vi "Main-Scanner.vi"() -> ()   [LabVIEW 2015]
uses:
  <vilib>/Utility/miscctls.llb/LVPointTypeDef.ctl
  <vilib>/Utility/sysdir.llb/System Directory Type.ctl
  <vilib>/event_ctls.llb/eventvkey.ctl
  <vilib>/Utility/config.llb/Read Key (I32).vi
  <vilib>/Utility/config.llb/Read Key (Boolean).vi
  <vilib>/Utility/config.llb/Read Key (String).vi
  <vilib>/Utility/config.llb/Write Key (U32).vi
  <vilib>/Utility/config.llb/Write Key (String).vi
  <vilib>/Utility/config.llb/NI_LVConfig.lvlib
panel:
  out "작업자명-Ready":bool=TRUE caption="Ready"
  out "Log 경로":path
  in  "Log File":bool
  out "공정단계-Ready":bool=TRUE caption="Ready"
  out "공정선택-Ready":bool=TRUE caption="Ready"
  out "Info.":string
  out "Ready":bool
  in  "제품번호":string
  in  "작업자명":string
  in  "공정 선택-Lock":bool caption="Lock"
  in  "공정단계":u16(ring) items=["Start", "Pass", "Fail"]
  in  "공정 선택":u16(ring) items=["Battery Cal.", "Glue Printing", "Leak Test", "FTS Test", "Package"]
  out "Path":path caption="경로 복제"
  out "ms 타이머 값":u32=30688000
  out "스캔 문자 삭제":bool=TRUE
  out "스캔 문자 수신 종료":bool
  out "Buf":string
  out "스캔 대기":bool=TRUE
  out "스캔 입력":bool
  in  "종료":bool=TRUE
  # "Ver. 161007"
  # "스캔대상"
  # "PCBA/박스.파우치"
  # "스캐너"
  # "Digital Scanner\n* DS4308"
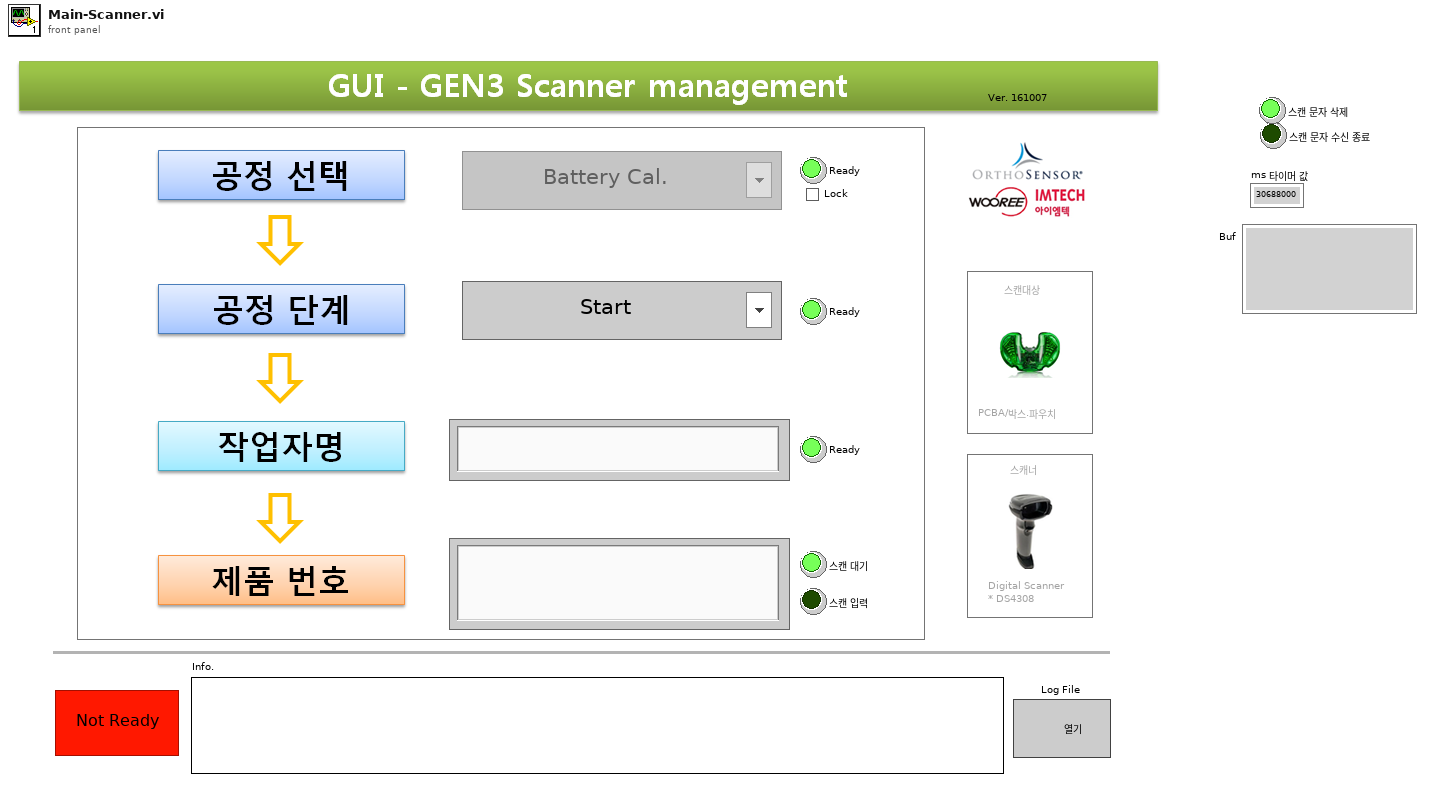
[diagram p1: front panel]
types:
  T1 = enum16{"Always On", "Always Off", "Off While Running"}
  T2 = typedef "LVPointTypeDef.ctl" = cluster{"Horizontal":i16, "Vertical":i16}
  T3 = enum8{"Enabled", "Disabled", "Disabled and Grayed Out"}
  T4 = typedef "eventvkey.ctl" = enum16{"ASCII", "Enter", "Return", "Shift", "Ctrl", "Alt", "Cmd", "Opt", "Caps", "NumLock", "Clear", "Break", "Up", "Down", "Left", "Right", "Insert", "Delete", "Home", "End", "PageUp", "PageDown", "Escape", "Help", "Pause", "ScrollLock", "F1", "F2", "F3", "F4", "F5", "F6", "F7", "F8", "F9", "F10", "F11", "F12", "F13", "F14", "F15", "F16", "F17", "F18", "F19", "F20", "F21", "F22", "F23", "F24", "Play", "VolumeUp", "VolumeDown", "Mute", "Two Byte Char"}
  T5 = enum16{"open", "replace", "create", "open or create", "replace or create", "replace or create with confirmation"}
  T6 = enum32{"invalid app kind", "Development System", "Run Time System", "Student Edition", "Embedded LabVIEW", "Evaluation", "Custom"}
  T7 = typedef "System Directory Type.ctl" = i32
  T8 = typedef "NI_LVConfig.lvlib/Config Data RefNum.ctl" = refnum<k1>
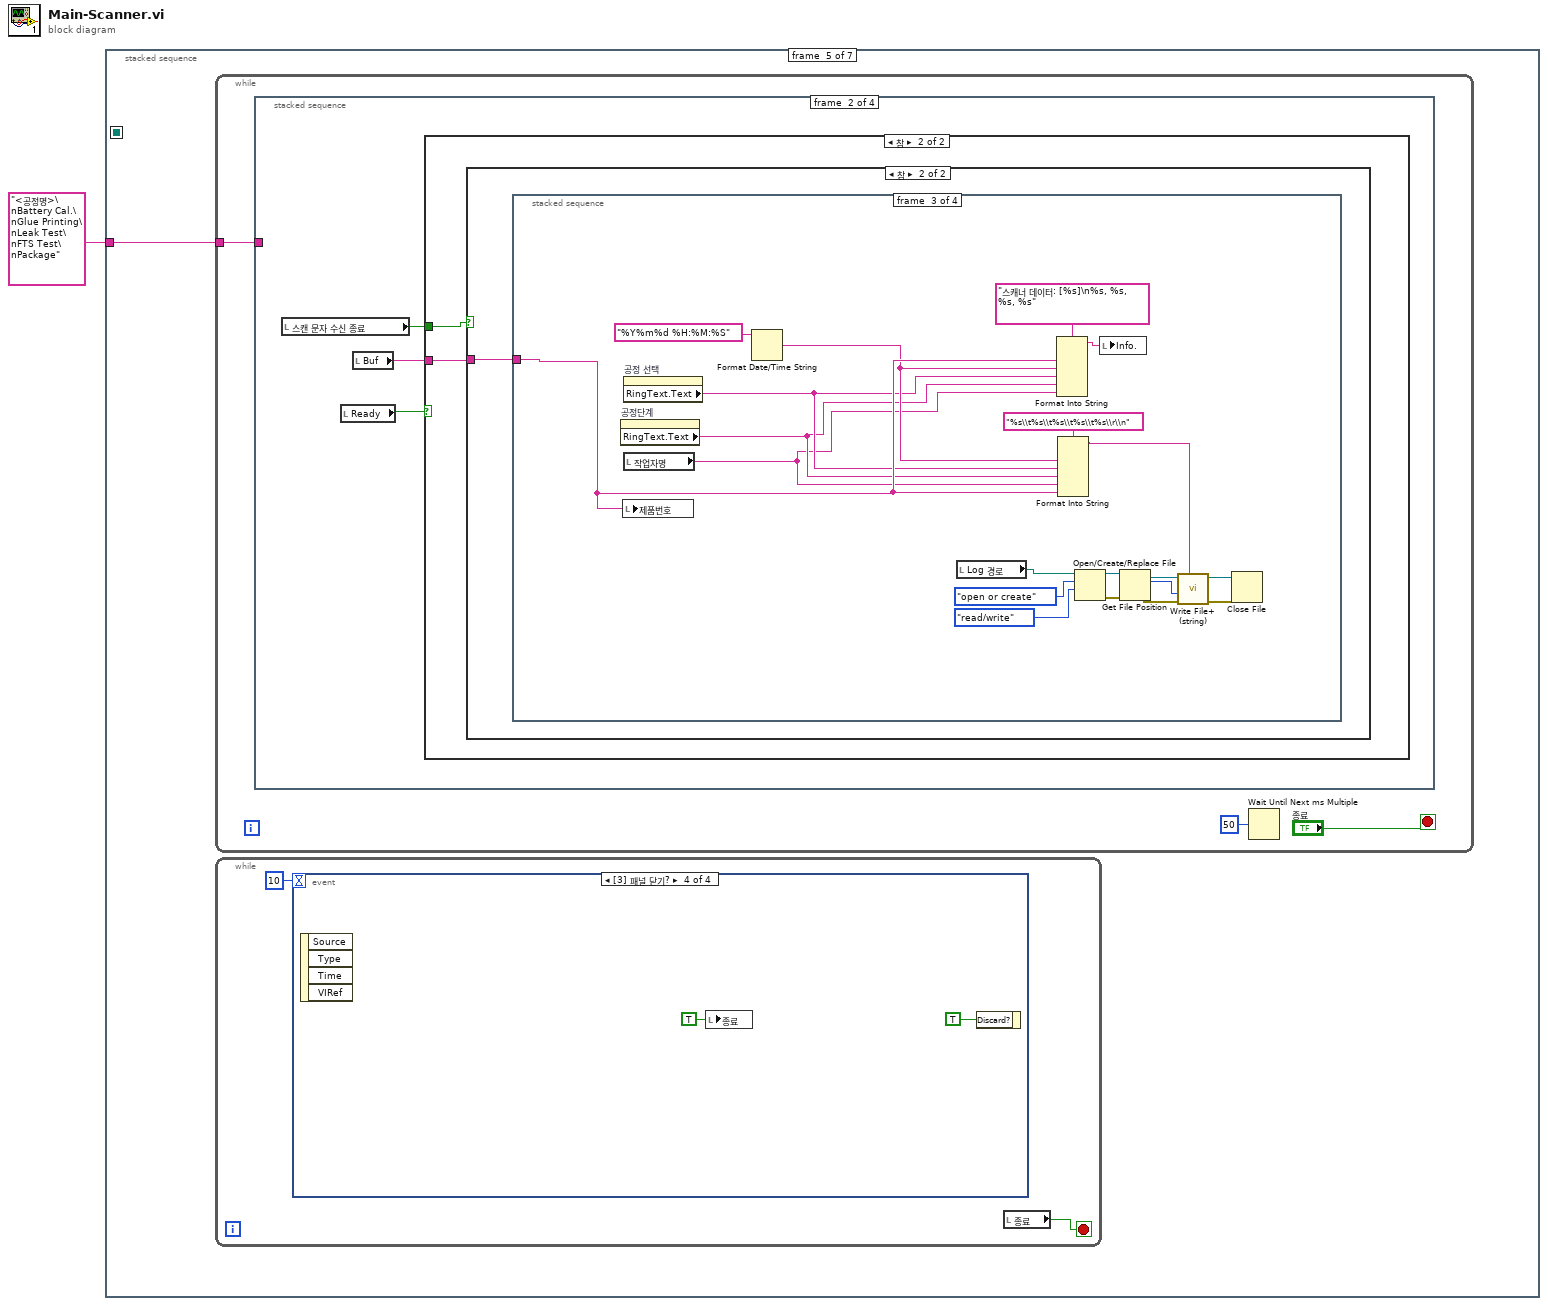
[diagram p0: block diagram]
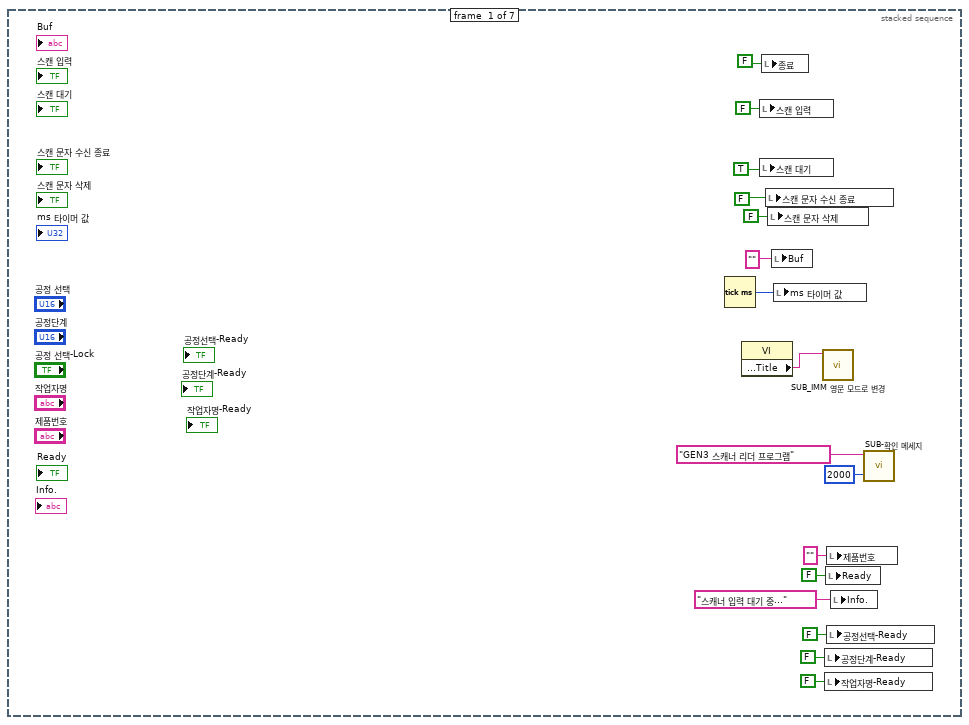
[diagram p2: hidden frame]
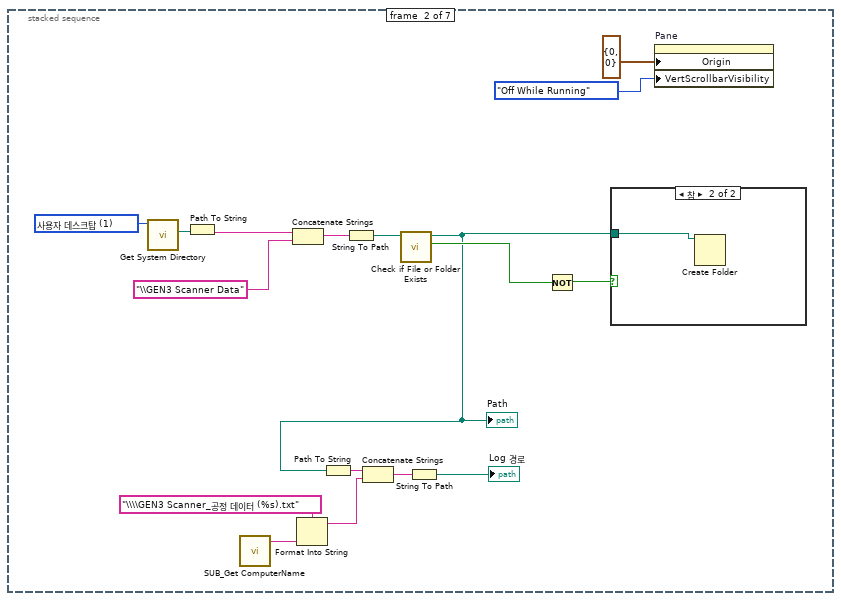
[diagram p3: hidden frame]
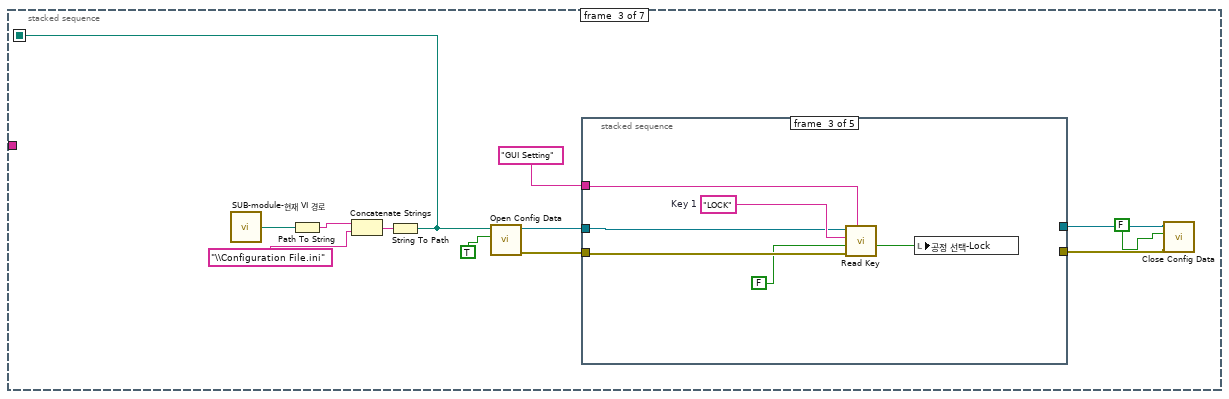
[diagram p5: hidden frame]
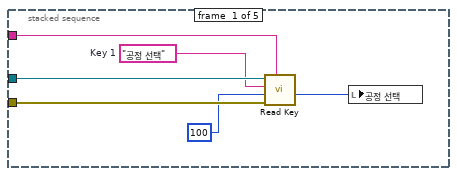
[diagram p6: hidden frame]
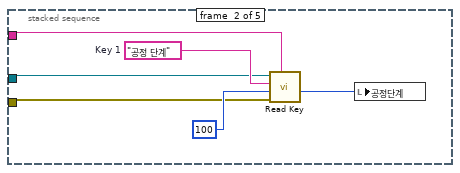
[diagram p7: hidden frame]
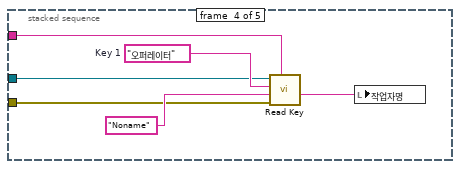
[diagram p8: hidden frame]
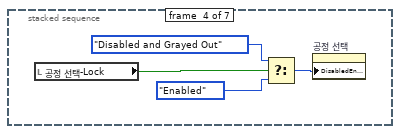
[diagram p10: hidden frame]
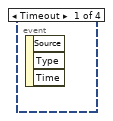
[diagram p11: hidden frame]
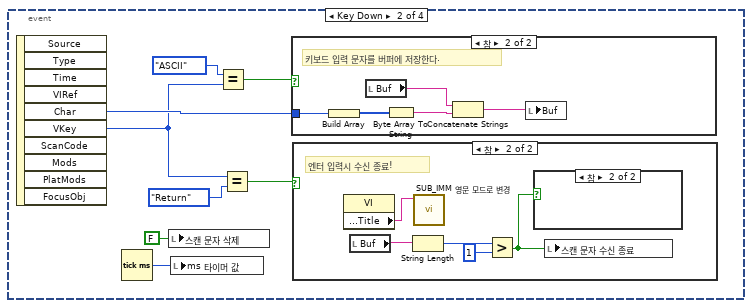
[diagram p12: hidden frame]
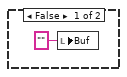
[diagram p14: hidden frame]
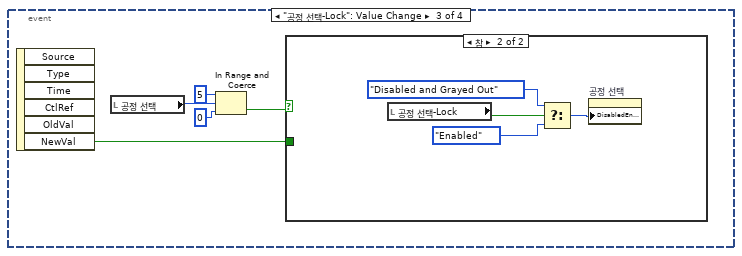
[diagram p16: hidden frame]
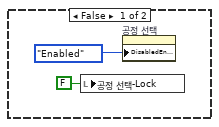
[diagram p17: hidden frame]
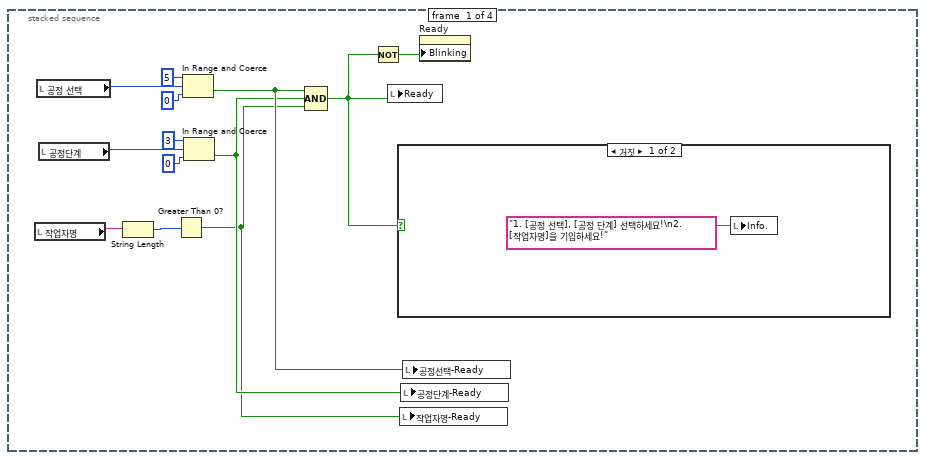
[diagram p18: hidden frame]
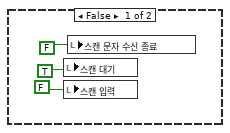
[diagram p20: hidden frame]
diagram:
  n1 = stacked-sequence {
    seq-local: [_ _ w36 _ _ _ _] -> [_ _ _ _ _ w179 _]
    tunnel: "<공정명>\nBattery Cal.\nGlue Printing\nLeak Test\nFTS Test\nPackage" ("공정 이름") -> [_ _ _ _ w78 _ _]
    frame #0 {
      n2 = Tick Count (ms)() -> (millisecond timer value=w15:u32)
      n3 = property class="VI"() -> ("Front Panel.Title"=w16:string)  [unwired: 2 in, 2 out]
      n4 = local write "스캔 입력"(FALSE ("스캔 종료")) -> ()
      n5 = local write "스캔 대기"(TRUE ("Clear")) -> ()
      n6 = local write "종료"(FALSE ("종료")) -> ()
      n7 = local write "스캔 문자 수신 종료"(FALSE ("스캔 종료")) -> ()
      n8 = local write "스캔 문자 삭제"(FALSE ("스캔 문자 삭제")) -> ()
      n9 = local write "Buf"("" ("스캐너 데이터")) -> ()
      n10 = local write "ms 타이머 값"(w15) -> ()
      n11 = call "SUB_IMM 영문 모드로 변경.vi"("프런트패널 윈도우:제목"=w16) -> ()  [unwired: 11 in]
      n12 = local write "공정단계-Ready"(FALSE ("공정선택-Ready")) -> ()
      n13 = local write "작업자명-Ready"(FALSE ("작업자명-Ready")) -> ()
      n14 = local write "Ready"(FALSE ("Ready")) -> ()
      n15 = local write "제품번호"("" ("제품번호")) -> ()
      n16 = local write "공정선택-Ready"(FALSE ("공정선택-Ready")) -> ()
      n17 = local write "Info."("스캐너 입력 대기 중..." ("Notice")) -> ()
      n18 = call "SUB-확인 메세지.vi"("타임아웃(ms)"=2000 ("타임아웃(s)"), "메세지"="GEN3 스캐너 리더 프로그램") -> ()  [unwired: 2 in]
    }
    frame #1 {
      w31 = T7 1 items=["사용자 홈"=0, "사용자 데스크탑"=1, "사용자 문서"=2, "사용자 어플리케이션 데이터"=3, "사용자 환경"=4, "사용자 임시"=5, "퍼블릭 문서"=6, "퍼블릭 어플리케이션 데이터"=7, "퍼블릭 환경"=8, "퍼블릭 캐시"=13, "시스템 코어 라이브러리"=9, "시스템 설치된 라이브러리"=10, "어플리케이션 파일"=11, "부팅 볼륨 루트"=12] ("system directory type")
      n19 = call <vilib>:"Get System Directory.vi"("system directory type"=w31) -> ("system directory"=w32:path)  [unwired: 10 in]
      n20 = Path To String(path=w32) -> (string=w30:string)
      n21 = call "SUB_Get ComputerName.vi"() -> ("String/Binary data"=w20:string)  [unwired: 4 in, 1 out]
      n22 = Concatenate Strings(w30, "\\GEN3 Scanner Data") -> (w28:string)
      n23 = Format Into String(format string="\\\\GEN3 Scanner_공정 데이터 (%s).txt" ("문자열"), w20) -> (resulting string=w22:string)  [unwired: 2 in, 1 out]
      n24 = String To Path(string=w28) -> (path=w27:path)
      n25 = call <vilib>:"Check if File or Folder Exists.vi"("path"=w27) -> ("file or folder exists?"=w25:bool, "dup path"=w19:path)  [unwired: 8 in, 1 out]
      "Path" <- w19
      n26 = Path To String(path=w19) -> (string=w24:string)
      n27 = Concatenate Strings(w24, w22) -> (w21:string)
      n28 = String To Path(string=w21) -> (path=→"Log 경로":path)
      n29 = Not(x=w25) -> (.not. x?=w26:bool)
      n30 = case shown="참" w26 {
        tunnel: w19 -> [_ w35]
        frame False {
        }
        frame True {
          n31 = Create Folder(path (use dialog)=w35) -> ()  [unwired: 2 in, 3 out]
        }
      }
      n32 = property on="Pane" class="Pane"("Origin"=T2 {"Horizontal"=0, "Vertical"=0} ("원점"), "VertScrollbarVisibility"=T1."Off While Running" ("수직 스크롤 막대 보이기")) -> ()  [unwired: 2 in, 2 out]
    }
    frame #2 {
      n33 = call "SUB-module-현재 VI 경로.vi"() -> ("현재 VI 경로"=w44:path)
      n34 = Path To String(path=w44) -> (string=w42:string)
      n35 = Concatenate Strings(w42, "\\Configuration File.ini") -> (w43:string)
      n36 = String To Path(string=w43) -> (path=w36:path)
      n37 = call <vilib>:"Open Config Data.vi"("create file if necessary (T)"=TRUE, "configuration file path"=w36) -> ("error out"=w38:errorcluster, "refnum"=w39:T8)  [unwired: 7 in, 1 out]
      n38 = stacked-sequence {
        tunnel: w39 -> [w53 w55 w62 w67 w73]
        tunnel: w38 -> [w52 w54 w61 w66 w72]
        tunnel: "GUI Setting" ("section") -> [w51 w56 w63 w68 _]
        tunnel: [_ _ _ _ w73] -> w46
        tunnel: [_ _ _ _ w72] -> w47
        frame #0 {
          w50 = "공정 선택"  # Key 1
          n39 = call-poly <vilib>:"Read Key.vi"("section"=w51, "error in (no error)"=w52, "default value"=100, "key"=w50, "refnum"=w53) -> ("value"=w49:i32)  [unwired: 3 in, 3 out]
          n40 = local write "공정 선택"(w49) -> ()
        }
        frame #1 {
          w59 = "공정 단계"  # Key 1
          n41 = call-poly <vilib>:"Read Key.vi"("section"=w56, "error in (no error)"=w54, "default value"=100, "key"=w59, "refnum"=w55) -> ("value"=w58:i32)  [unwired: 3 in, 3 out]
          n42 = local write "공정단계"(w58) -> ()
        }
        frame #2 {
          w65 = "LOCK"  # Key 1
          n43 = call-poly <vilib>:"Read Key.vi"("section"=w63, "error in (no error)"=w61, "default value"=FALSE, "key"=w65, "refnum"=w62) -> ("value"=w64:bool)  [unwired: 3 in, 3 out]
          n44 = local write "공정 선택-Lock"(w64) -> ()
        }
        frame #3 {
          w71 = "오퍼레이터"  # Key 1
          n45 = call-poly <vilib>:"Read Key.vi"("section"=w68, "error in (no error)"=w66, "default value"="Noname" ("section"), "key"=w71, "refnum"=w67) -> ("value"=w70:string)  [unwired: 3 in, 3 out]
          n46 = local write "작업자명"(w70) -> ()
        }
        frame #4 {
        }
      }
      n47 = call <vilib>:"Close Config Data.vi"("error in (no error)"=w47, "write file if changed (T)"=FALSE ("write configuration file? (T)"), "refnum"=w46) -> ()  [unwired: 9 out]
    }
    frame #3 {
      n48 = local read "공정 선택-Lock"() -> (w77:bool)
      n49 = Select(t=T3."Disabled and Grayed Out" ("비활성화"), s=w77, f=T3."Enabled" ("비활성화")) -> (s? t:f=w74:T3)
      n50 = property on="공정 선택" class="Ring (엄격한)"("DisabledEnum"=w74) -> ()  [unwired: 2 in, 2 out]
    }
    frame #4 {
      n51 = while {
        tunnel: w78 -> [w113]
        stop <- "종료" stop-if-true
        n52 = stacked-sequence {
          tunnel: w113 -> [_ _ _ _]
          frame #0 {
            n53 = local read "작업자명"() -> (w118:string)
            n54 = local read "공정 선택"() -> (w128:u16)
            n55 = local read "공정단계"() -> (w123:u16)
            n56 = String Length(string=w118) -> (length=w117:i32)
            n57 = Greater Than 0?(x=w117) -> (x > 0?=w116:bool)
            n58 = In Range and Coerce(upper limit=u16 5 ("상위 리미트"), x=w128, lower limit=u16 0 ("상위 리미트")) -> (In Range?=w120:bool)  [unwired: 1 out]
            n59 = In Range and Coerce(upper limit=u16 3 ("상위 리미트"), x=w123, lower limit=u16 0 ("상위 리미트")) -> (In Range?=w119:bool)  [unwired: 1 out]
            n60 = Compound Arithmetic op=AND ("복합 연산")(w120, w119, w116) -> (w121:bool)
            n61 = Not(x=w121) -> (.not. x?=w122:bool)
            n62 = local write "Ready"(w121) -> ()
            n63 = case shown="거짓" w121 {
              frame False {
                n64 = local write "Info."("1. [공정 선택], [공정 단계] 선택하세요!\n2. [작업자명]을 기입하세요!" ("Notice")) -> ()
              }
              frame True {
              }
            }
            n65 = local write "작업자명-Ready"(w116) -> ()
            n66 = local write "공정단계-Ready"(w119) -> ()
            n67 = local write "공정선택-Ready"(w120) -> ()
            n68 = property on="Ready" class="Bool (엄격한)"("Blinking"=w122) -> ()  [unwired: 2 in, 2 out]
          }
          frame #1 {
            n69 = local read "스캔 문자 수신 종료"() -> (w131:bool)
            n70 = local read "Ready"() -> (w132:bool)
            n71 = local read "Buf"() -> (w130:string)
            n72 = case shown="참" w132 {
              tunnel: w131 -> [_ w137]
              tunnel: w130 -> [_ w136]
              frame False {
                n73 = local write "스캔 대기"(TRUE ("Clear")) -> ()
                n74 = local write "스캔 입력"(FALSE ("스캔 종료")) -> ()
                n75 = local write "스캔 문자 수신 종료"(FALSE ("스캔 종료")) -> ()
              }
              frame True {
                n76 = case shown="참" w137 {
                  tunnel: w136 -> [_ w138]
                  frame False {
                  }
                  frame True {
                    n77 = stacked-sequence {
                      tunnel: w138 -> [_ _ w149 _]
                      frame #0 {
                        n78 = local write "스캔 대기"(FALSE ("Clear")) -> ()
                        n79 = local write "스캔 입력"(TRUE ("스캔 종료")) -> ()
                        n80 = local write "제품번호"("" ("제품번호")) -> ()
                        n81 = local write "Info."("" ("Notice")) -> ()
                      }
                      frame #1 {
                        n82 = Wait (ms)(milliseconds to wait=u32 250 ("대기 시간(ms)")) -> ()  [unwired: 1 out]
                      }
                      frame #2 {
                        n83 = property on="공정단계" class="Ring (엄격한)"() -> ("RingText.Text"=w146:string)  [unwired: 2 in, 2 out]
                        n84 = local write "제품번호"(w149) -> ()
                        n85 = property on="공정 선택" class="Ring (엄격한)"() -> ("RingText.Text"=w147:string)  [unwired: 2 in, 2 out]
                        n86 = local read "작업자명"() -> (w145:string)
                        n87 = Format Date/Time String(time format string (%c)="%Y%m%d %H:%M:%S" ("시간 포맷 문자열 (%c)")) -> (date/time string=w148:string)  [unwired: 2 in]
                        n88 = local read "Log 경로"() -> (w144:path)
                        n89 = Format Into String(format string="스캐너 데이터: [%s]\n%s, %s, %s, %s" ("포맷 문자열"), w149, w148, w147, w146, w145) -> (resulting string=w151:string)  [unwired: 2 in, 1 out]
                        n90 = Format Into String(format string="%s\\t%s\\t%s\\t%s\\t%s\\r\\n" ("포맷 문자열"), w148, w147, w146, w145, w149) -> (resulting string=w152:string)  [unwired: 2 in, 1 out]
                        n91 = Open/Create/Replace File(file path (use dialog)=w144, operation (0:open)=T5."open or create" ("동작(0:open)"), access (0:read/write)=enum16{"read/write", "read-only", "write-only"}."read/write" ("접근(0:읽기/쓰기)")) -> (refnum out=w159:refnum<file>, error out=w160:errorcluster)  [unwired: 3 in, 1 out]
                        n92 = local write "Info."(w151) -> ()
                        n93 = Get File Position(4:w160, 7:w159) -> (0:w156:errorcluster, 2:w161:i64, 3:w155:refnum<file>)
                        n94 = call <vilib>:"Write File+ (string).vi"("string"=w152, "error in (no error)"=w156, "pos offset (bytes:0)"=w161, "refnum"=w155) -> ("error out"=w154:errorcluster, "dup refnum"=w162:refnum<file>)  [unwired: 3 in, 1 out]
                        n95 = Close File(refnum=w162, error in=w154) -> ()  [unwired: 2 out]
                      }
                      frame #3 {
                        n96 = local write "스캔 대기"(TRUE ("Clear")) -> ()
                        n97 = local write "스캔 입력"(FALSE ("스캔 종료")) -> ()
                        n98 = local write "Buf"("" ("스캐너 데이터")) -> ()
                        n99 = local write "스캔 문자 수신 종료"(FALSE ("스캔 종료")) -> ()
                      }
                    }
                  }
                }
              }
            }
          }
          frame #2 {
            # "스캐너 문자열 타임아웃"
            n100 = local read "ms 타이머 값"() -> (w170:u32)
            n101 = Tick Count (ms)() -> (millisecond timer value=w169:u32)
            n102 = Subtract(x=w169, y=w170) -> (x-y=w168:u32)
            n103 = case shown="200.." w168 {
              frame 0, Default {
              }
              frame 200.. {
                n104 = Tick Count (ms)() -> (millisecond timer value=w172:u32)
                n105 = local write "스캔 문자 삭제"(TRUE ("스캔 문자 삭제")) -> ()
                n106 = local write "ms 타이머 값"(w172) -> ()
                n107 = local write "Buf"("" ("스캐너 데이터")) -> ()
              }
            }
          }
          frame #3 {
            n108 = case shown="참" "Log File" {
              frame False {
              }
              frame True {
                n109 = local read "Log 경로"() -> (w175:path)
                n110 = Format Into String(format string="Notepad.exe %s", w175) -> (resulting string=w177:string)  [unwired: 2 in, 1 out]
                n111 = call <vilib>:"System Exec.vi"("wait until completion? (T)"=FALSE, "command line"=w177) -> ()  [unwired: 4 in, 6 out]
              }
            }
          }
        }
        n112 = Wait Until Next ms Multiple(millisecond multiple=u32 50) -> ()  [unwired: 1 out]
      }
      n113 = while {
        stop <- w80 stop-if-true
        n114 = event shown="[3] 패널 닫기?" {
          selector: _ -> [_ _ _ _]
          dyn-events: _ -> [_ _ _ _]
          timeout: 10 -> [_ _ _ _]
          event Timeout {
            n115 = event-data() -> ()  [unwired: 1 in, 3 out]
          }
          event Key Down {
            n116 = event-data() -> ("Char"=w86:i16, "VKey"=w84:T4)  [unwired: 1 in, 8 out]
            n117 = Tick Count (ms)() -> (millisecond timer value=w82:u32)
            n118 = local write "스캔 문자 삭제"(FALSE ("스캔 문자 삭제")) -> ()
            n119 = local write "ms 타이머 값"(w82) -> ()
            n120 = Equal?(x=eventvkey."ASCII" ("V 키"), y=w84) -> (x = y?=w88:bool)
            n121 = Equal?(x=w84, y=eventvkey."Return" ("V 키")) -> (x = y?=w83:bool)
            n122 = case shown="참" w88 {
              tunnel: w86 -> [_ w99]
              frame False {
              }
              frame True {
                # "키보드 입력 문자를 버퍼에 저장한다."
                n123 = Build Array(w99) -> (w98:i16[])
                n124 = local read "Buf"() -> (w97:string)
                n125 = Byte Array To String(unsigned byte array=w98) -> (string=w96:string)
                n126 = Concatenate Strings(w97, w96) -> (w95:string)
                n127 = local write "Buf"(w95) -> ()
              }
            }
            n128 = case shown="참" w83 {
              frame False {
              }
              frame True {
                # "엔터 입력시 수신 종료!"
                n129 = property class="VI"() -> ("Front Panel.Title"=w93:string)  [unwired: 2 in, 2 out]
                n130 = local read "Buf"() -> (w92:string)
                n131 = String Length(string=w92) -> (length=w91:i32)
                n132 = call "SUB_IMM 영문 모드로 변경.vi"("프런트패널 윈도우:제목"=w93) -> ()  [unwired: 11 in]
                n133 = Greater?(x=w91, y=1) -> (0:w89:bool)
                n134 = case shown="참" w89 {
                  frame False {
                    n135 = local write "Buf"("" ("Buf")) -> ()
                  }
                  frame True {
                  }
                }
                n136 = local write "스캔 문자 수신 종료"(w89) -> ()
              }
            }
          }
          event "공정 선택-Lock": Value Change {
            n137 = event-data() -> ("NewVal"=w100:bool)  [unwired: 1 in, 5 out]
            n138 = local read "공정 선택"() -> (w102:u16)
            n139 = In Range and Coerce(upper limit=u16 5 ("상위 리미트"), x=w102, lower limit=u16 0 ("상위 리미트")) -> (In Range?=w101:bool)  [unwired: 1 out]
            n140 = case shown="참" w101 {
              tunnel: w100 -> [_ _]
              frame False {
                n141 = local write "공정 선택-Lock"(FALSE ("공정 선택-Lock")) -> ()
                n142 = property on="공정 선택" class="Ring (엄격한)"("DisabledEnum"=T3."Enabled" ("비활성화")) -> ()  [unwired: 2 in, 2 out]
              }
              frame True {
                n143 = local read "공정 선택-Lock"() -> (w110:bool)
                n144 = Select(t=T3."Disabled and Grayed Out" ("비활성화"), s=w110, f=T3."Enabled" ("비활성화")) -> (s? t:f=w107:T3)
                n145 = property on="공정 선택" class="Ring (엄격한)"("DisabledEnum"=w107) -> ()  [unwired: 2 in, 2 out]
              }
            }
          }
          event Panel Close? {
            n146 = event-data() -> ()  [unwired: 1 in, 4 out]
            n147 = local write "종료"(TRUE ("종료")) -> ()
            n148 = event-data("Discard?"=TRUE ("버림?")) -> ()  [unwired: 1 in, 1 out]
          }
        }
        n149 = local read "종료"() -> (w80:bool)
      }
    }
    frame #5 {
      n150 = call <vilib>:"Open Config Data.vi"("configuration file path"=w179) -> ("error out"=w184:errorcluster, "refnum"=w183:T8)  [unwired: 2 in, 7 out]
      n151 = stacked-sequence {
        tunnel: w183 -> [w186 w191 w196 w201 w206]
        tunnel: w184 -> [w185 w190 w195 w200 w205]
        tunnel: "GUI Setting" ("section") -> [w187 w192 w197 w202 _]
        tunnel: [_ _ _ _ w206] -> w181
        tunnel: [_ _ _ _ w205] -> w180
        frame #0 {
          w189 = "공정 선택"  # Key 1
          n152 = local read "공정 선택"() -> (w188:u16)
          n153 = call-poly <vilib>:"Write Key.vi"("section"=w187, "error in (no error)"=w185, "value"=w188, "key"=w189, "refnum"=w186) -> ()  [unwired: 7 out]
        }
        frame #1 {
          w194 = "공정 단계"  # Key 1
          n154 = local read "공정단계"() -> (w193:u16)
          n155 = call-poly <vilib>:"Write Key.vi"("section"=w192, "error in (no error)"=w190, "value"=w193, "key"=w194, "refnum"=w191) -> ()  [unwired: 7 out]
        }
        frame #2 {
          w199 = "공정 단계"  # Key 1
          n156 = local read "공정단계"() -> (w198:u16)
          n157 = call-poly <vilib>:"Write Key.vi"("section"=w197, "error in (no error)"=w195, "value"=w198, "key"=w199, "refnum"=w196) -> ()  [unwired: 7 out]
        }
        frame #3 {
          w204 = "오퍼레이터"  # Key 1
          n158 = local read "작업자명"() -> (w203:string)
          n159 = call-poly <vilib>:"Write Key.vi"("section"=w202, "error in (no error)"=w200, "value"=w203, "key"=w204, "refnum"=w201) -> ()  [unwired: 1 in, 6 out]
        }
        frame #4 {
        }
      }
      n160 = call <vilib>:"Close Config Data.vi"("error in (no error)"=w180, "refnum"=w181) -> ()  [unwired: 1 in, 9 out]
    }
    frame #6 {
      # "exe 실행 파일인 경우에는 완전 종료"
      n161 = property class="App"() -> ("App.Kind"=w208:T6)  [unwired: 2 in, 2 out]
      n162 = Equal?(x=w208, y=T6."Run Time System" ("Application:Kind")) -> (x = y?=w207:bool)
      n163 = Quit LabVIEW(quit? (T)=w207) -> ()
    }
  }
